vi "SetDuration.vi"(8 "error in (no error)":errorcluster, 9 "Duration [s]":dbl, 10 "Tag Name":string, 11 "ResultTree in":refnum<class "ResultTree.lvclass">) -> (0 "error out":errorcluster, 3 "ResultTree out":refnum<class "ResultTree.lvclass">)   [LabVIEW 2017, in "ResultTree.lvclass"]
doc: "Sets the duration. <B>Duration</B> must be specified in <B>seconds</B>."
uses:
  ResultTree.lvclass
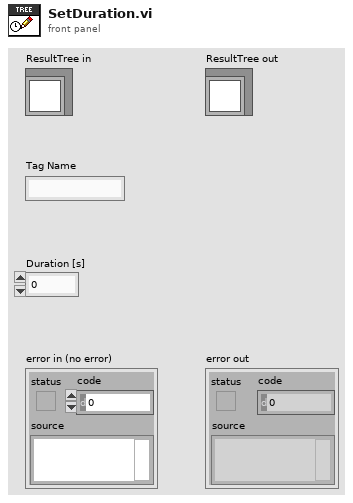
[diagram p1: front panel]
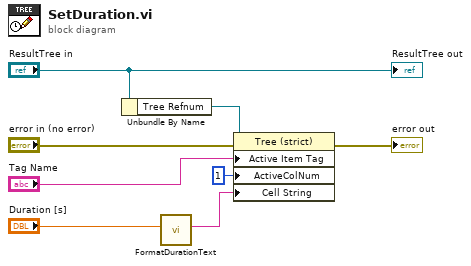
[diagram p0: block diagram]
diagram:
  n1 = Unbundle By Name("ResultTree in") -> ("Tree Refnum"=w4:refnum<vi>)
  n2 = call "FormatDurationText.vi"("Duration [s]"="Duration [s]") -> ("String"=w1:string)  [unwired: 10 in]
  n3 = property class="Tree (strict)"(reference=w4, error in="error in (no error)", "Active Item Tag"="Tag Name", "ActiveColNum"=1 ("Active Cell:Active Column Number"), "Cell String"=w1) -> (error out=→"error out":errorcluster)  [unwired: 1 out]
  "ResultTree out" <- "ResultTree in"
